vi "Permutation solution.vi"() -> ()   [LabVIEW 2018]
uses:
  ctl/Coin data--cluster.ctl
  ctl/Comparison result--enum.ctl
  <userlib>/_OpenG.lib/array/array.llb/Reverse 2D Array (Boolean)__ogtk.vi
panel:
  out "Result":string
  out "Finished message":string
  out "Goal amount":dbl=7.0 format="£%#_g"
  out "No. solutions found":i32
  out "Total left in tree":dbl format="£%.2g"
  in  "Stop":bool
  out "Total of coins selected":dbl format="£%#.2g"
  out "Coins":bool[](array[boolean])
  out "Solutions found":bool[][](array[boolean])
  # "Beer Money"
  # "Permutation Solution"
  # "What's going on?\n\nThe algorithm is doing a breadth first search of the tree.\n\nIf the result is below the goal amount, it adds it to a list to come back to later. If the result is above the goal amount, it moves the lowest value coin to the next smallest denomination.\n\nIt is seriously slow - you won't get to the end unless you have a supercomputer. Make use of the stop button.\n\nTheoretically it can check every permutation and it finds the correct solution for smaller problems."
  # "1p"
  # "2p"
  # "5p"
  # "10p"
  # "20p"
  # "50p"
  # "£1"
  # "£2"
  # "£5"
  # "£10"
  # "Link to better explanation:\n\nhttps://youtu.be/z-Rf1_xs25s"
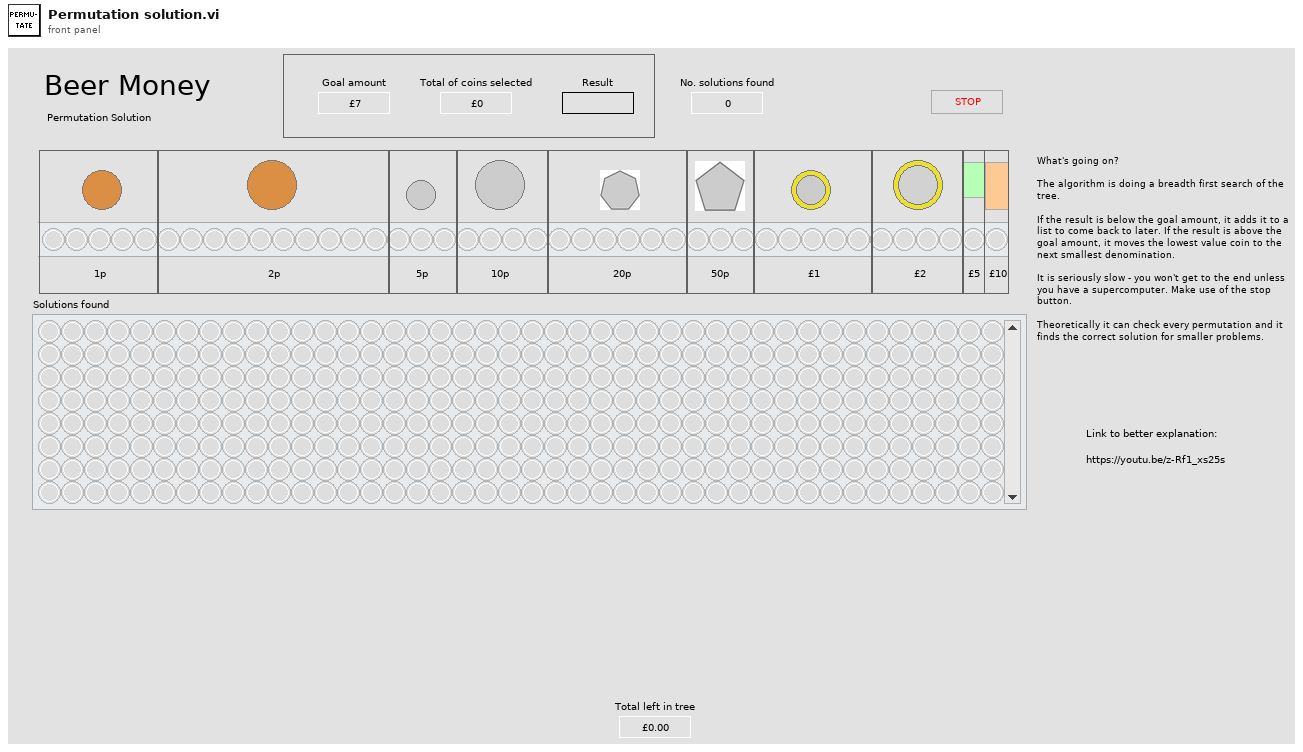
[diagram p1: front panel]
types:
  T1 = typedef "Coin data--cluster.ctl" = cluster{"Coin/note":i32, "Quantity":i32}
  T2 = cluster{"Wallet contents":T1[], "All my coins (values, £)":dbl[], "Indexes of next denom":i32[], "Wallet total (£)":dbl, "Index":i32, "Goal amount (£)":dbl, "No. coins":i32, "Coins State Cache":bool[], "Successful combos":bool[][], "'Hold' list (unexplored)":bool[][]}
  T3 = typedef "Comparison result--enum.ctl" = enum16{"Under", "Bingo!", "Over"}
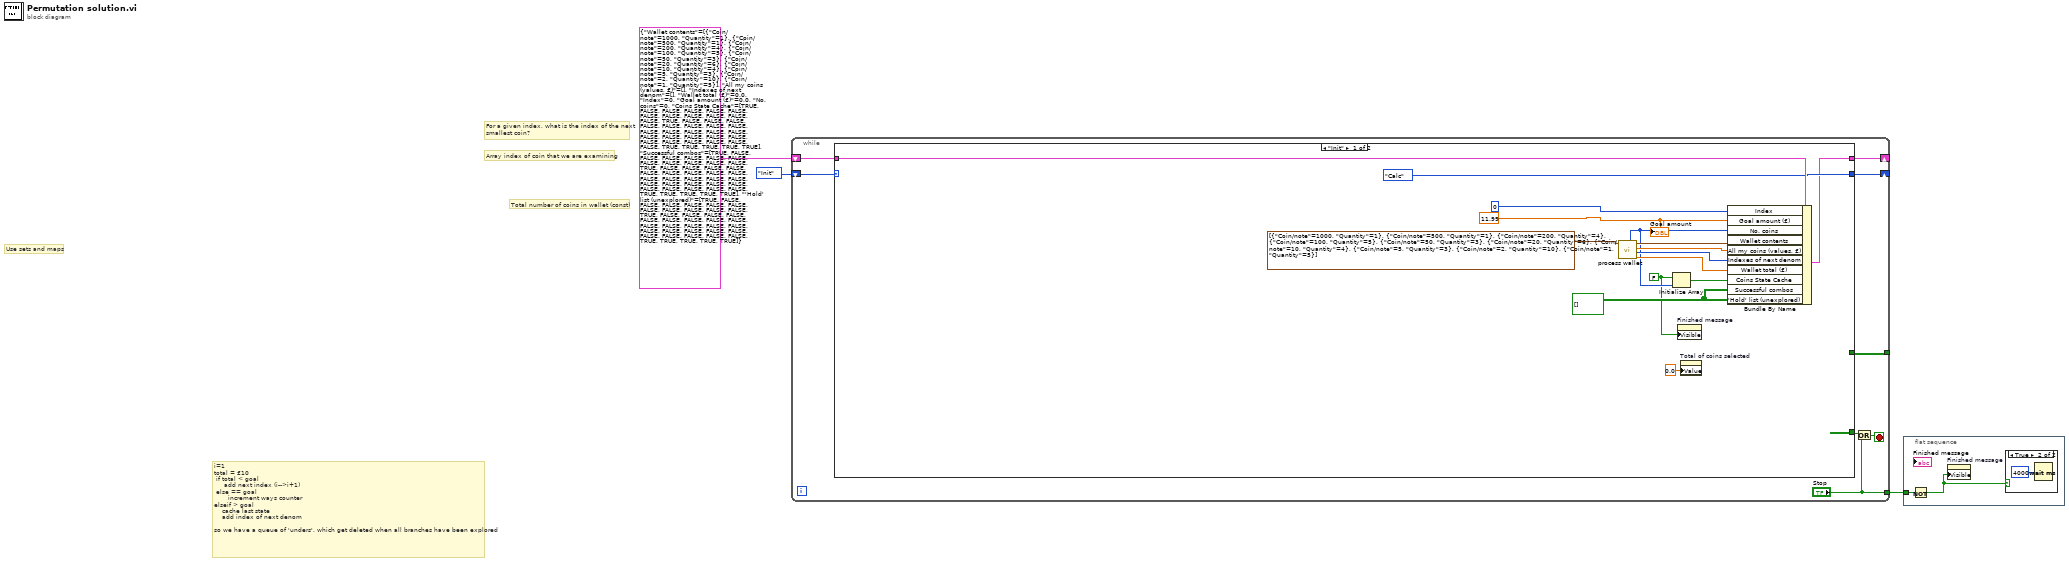
[diagram p0: block diagram]
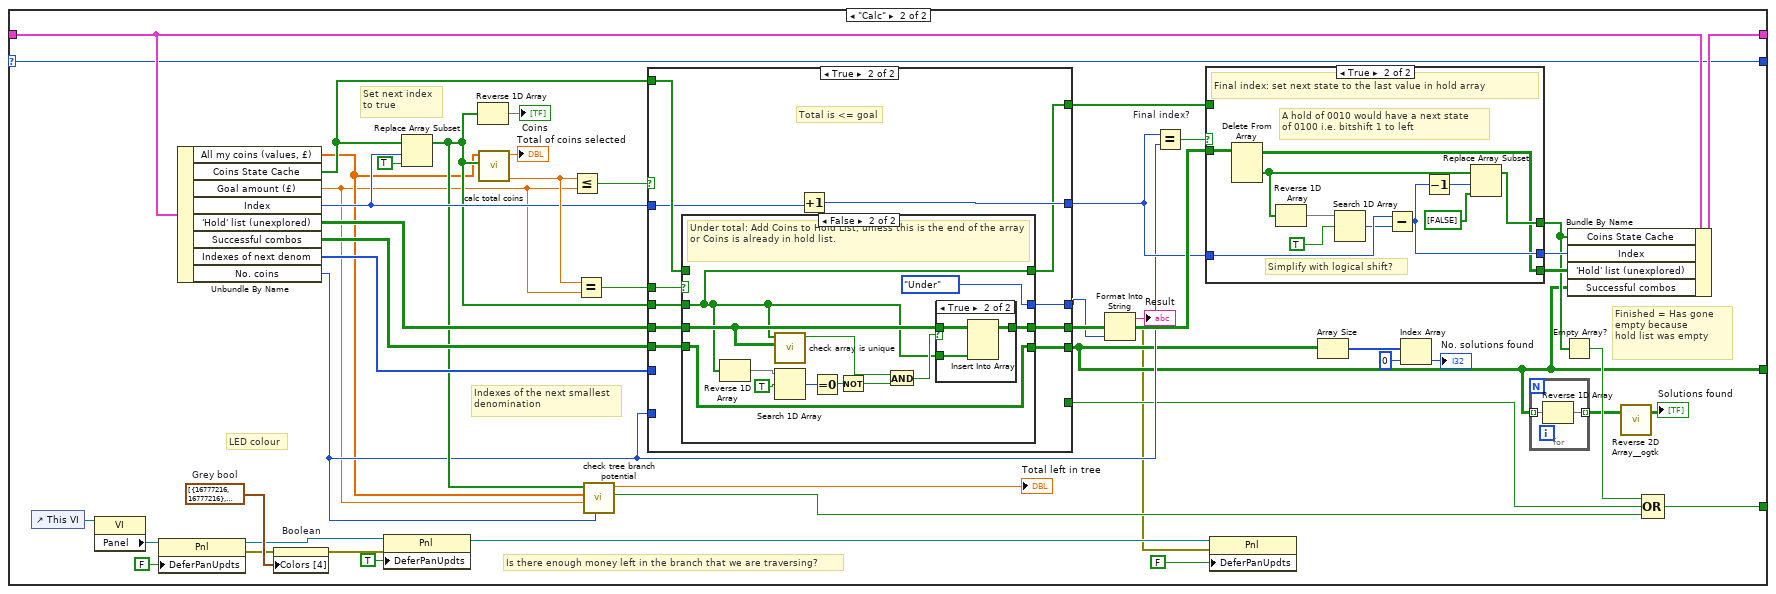
[diagram p3: hidden frame]
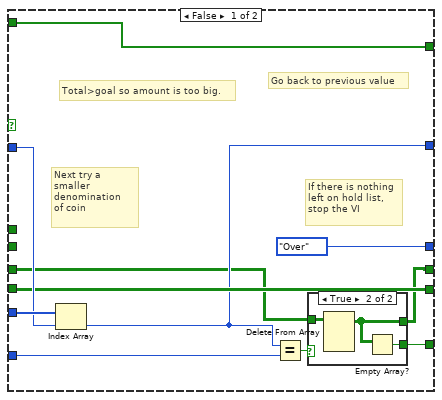
[diagram p5: hidden frame]
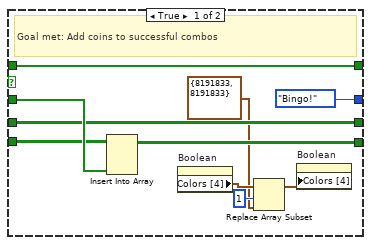
[diagram p7: hidden frame]
diagram:
  # "For a given index, what is the index of the next\nsmallest coin?"
  # "Total number of coins in wallet (const)"
  # "Array index of coin that we are examining"
  # "i=1\ntotal = £10\n if total < goal\n     add next index (i-->i+1)\n else == goal\n       increment ways counter\nelseif > goal\n    cache last state\n    add index of next denom\n\nso we have a queue of 'unders', which get deleted when all branches have been explored"
  # "Use sets and maps"
  n1 = while {
    shift-right: [w10] -> _
    shift-left: T2 {"Wallet contents"=[{"Coin/note"=1000, "Quantity"=1}, {"Coin/note"=500, "Quantity"=1}, {"Coin/note"=200, "Quantity"=4}, {"Coin/note"=100, "Quantity"=5}, {"Coin/note"=50, "Quantity"=3}, {"Coin/note"=20, "Quantity"=6}, {"Coin/note"=10, "Quantity"=4}, {"Coin/note"=5, "Quantity"=3}, {"Coin/note"=2, "Quantity"=10}, {"Coin/note"=1, "Quantity"=5}], "All my coins (values, £)"=[], "Indexes of next denom"=[], "Wallet total (£)"=0.0, "Index"=0, "Goal amount (£)"=0.0, "No. coins"=0, "Coins State Cache"=[TRUE, FALSE, FALSE, FALSE, FALSE, FALSE, FALSE, FALSE, FALSE, FALSE, FALSE, FALSE, TRUE, FALSE, FALSE, FALSE, FALSE, FALSE, FALSE, FALSE, FALSE, FALSE, FALSE, FALSE, FALSE, FALSE, FALSE, FALSE, FALSE, FALSE, FALSE, FALSE, FALSE, FALSE, FALSE, FALSE, FALSE, TRUE, TRUE, TRUE, TRUE, TRUE], "Successful combos"=[[TRUE, FALSE, FALSE, FALSE, FALSE, FALSE, FALSE, FALSE, FALSE, FALSE, FALSE, FALSE, TRUE, FALSE, FALSE, FALSE, FALSE, FALSE, FALSE, FALSE, FALSE, FALSE, FALSE, FALSE, FALSE, FALSE, FALSE, FALSE, FALSE, FALSE, FALSE, FALSE, FALSE, FALSE, FALSE, FALSE, FALSE, TRUE, TRUE, TRUE, TRUE, TRUE]], "'Hold' list (unexplored)"=[[TRUE, FALSE, FALSE, FALSE, FALSE, FALSE, FALSE, FALSE, FALSE, FALSE, FALSE, FALSE, TRUE, FALSE, FALSE, FALSE, FALSE, FALSE, FALSE, FALSE, FALSE, FALSE, FALSE, FALSE, FALSE, FALSE, FALSE, FALSE, FALSE, FALSE, FALSE, FALSE, FALSE, FALSE, FALSE, FALSE, FALSE, TRUE, TRUE, TRUE, TRUE, TRUE]]} -> [w11]
    shift-right: [w8] -> _
    shift-left: enum16{"Init", "Calc"}."Init" -> [w9]
    tunnel: [w6] -> _
    tunnel: ["Stop"] -> w1
    stop <- w5 stop-if-true
    n2 = case shown="\"Init\"" w9 {
      selector: w9 -> [_ w66]
      tunnel: w11 -> [w26 w73]
      tunnel: [w16 w74] -> w10
      tunnel: [_ w49] -> w7
      tunnel: [enum16{"Init", "Calc"}."Calc" w66] -> w8
      tunnel: [_ w43] -> w6
      frame "Init" {
        w14 = FALSE
        w23 = 11.99 ("goal amount")
        w25 = bool[][] [] ("'Hold' list (unexplored)")
        n3 = call "process wallet.vi"("Wallet contents"=T1[] [{"Coin/note"=1000, "Quantity"=1}, {"Coin/note"=500, "Quantity"=1}, {"Coin/note"=200, "Quantity"=4}, {"Coin/note"=100, "Quantity"=5}, {"Coin/note"=50, "Quantity"=3}, {"Coin/note"=20, "Quantity"=6}, {"Coin/note"=10, "Quantity"=4}, {"Coin/note"=5, "Quantity"=3}, {"Coin/note"=2, "Quantity"=10}, {"Coin/note"=1, "Quantity"=5}]) -> ("Wallet total (£)"=w19:dbl, "Indexes of next denom"=w20:i32[], "All my coins (values, £)"=w21:dbl[], "Wallet contents (dup)"=w22:T1[], "No. coins"=w15:i32)  [unwired: 6 in]
        n4 = Initialize Array(w14, w15) -> (w18:bool[])
        n5 = property on="Finished message" class="Str"("Visible"=w14) -> ()  [unwired: 2 in, 2 out]
        n6 = property on="Total of coins selected" class="DigNum (strict)"("Value"=0.0 ("Total of coins selected")) -> ()  [unwired: 2 in, 2 out]
        n7 = Bundle By Name(cluster=w26, "Index"=0, "Goal amount (£)"=w23, "No. coins"=w15, "Wallet contents"=w22, "All my coins (values, £)"=w21, "Indexes of next denom"=w20, "Wallet total (£)"=w19, "Coins State Cache"=w18, "Successful combos"=w25, "'Hold' list (unexplored)"=w25) -> (w16:T2)
        "Goal amount" <- w23
      }
      frame "Calc" {
        w39 = cluster{u32, u32}[] [{16777216, 16777216}, {8026746, 8026746}, {16777216, 16777216}, {4095788, 4095788}]  # Grey bool
        # "LED colour"
        # "Indexes of the next smallest\ndenomination"
        # "Is there enough money left in the branch that we are traversing?"
        # "Set next index to true"
        # "Finished = Has gone empty because\nhold list was empty"
        n8 = control-ref of="This VI"() -> (w37:refnum<vi>)
        n9 = property class="VI"(reference=w37) -> ("Panel"=w36:refnum<vi>)  [unwired: 1 in, 2 out]
        n10 = property class="Pnl"(reference=w36, "DeferPanUpdts"=FALSE ("Defer Panel Updates")) -> (reference out=w33:refnum<vi>, error out=w30:errorcluster)  [unwired: 1 in]
        n11 = Unbundle By Name(w73) -> ("All my coins (values, £)"=w52:dbl[], "Coins State Cache"=w55:bool[], "Goal amount (£)"=w50:dbl, "Index"=w62:i32, "'Hold' list (unexplored)"=w69:bool[][], "Successful combos"=w68:bool[][], "Indexes of next denom"=w67:i32[], "No. coins"=w53:i32)
        n12 = property on="Boolean" class="Bool (strict)"(error in=w30, "Colors [4]"=w39) -> (error out=w32:errorcluster)  [unwired: 1 in, 1 out]
        n13 = property class="Pnl"(reference=w33, error in=w32, "DeferPanUpdts"=TRUE ("Defer Panel Updates")) -> (reference out=w29:refnum<vi>)  [unwired: 1 out]
        n14 = Replace Array Subset(array=w55, new element=TRUE ("new element/subarray"), index=w62) -> (w54:bool[])
        n15 = Reverse 1D Array(array=w54) -> (reversed array=→"Coins":bool[])
        n16 = call "calc total coins.vi"("Coins"=w54, "All my coins"=w52) -> ("Total (£)"=w71:dbl)  [unwired: 9 in]
        "Total of coins selected" <- w71
        n17 = Less Or Equal?(x=w71, y=w50) -> (x <= y?=w72:bool)
        n18 = Equal?(x=w71, y=w50) -> (x = y?=w70:bool)
        n19 = call "check tree branch potential.vi"("No. coins"=w53, "Goal amount"=w50, "All my coins"=w52, "Coins State Cache"=w54) -> ("Stop?"=w48:bool, "Total (£)"=→"Total left in tree":dbl)  [unwired: 6 in]
        n20 = case "Goal amount exceeded?" shown="True" w72 {
          tunnel: w70 -> [_ w106]
          tunnel: w62 -> [w100 w107]
          tunnel: [w96 w116] -> w59
          tunnel: w54 -> [_ w112]
          tunnel: w69 -> [w95 w115]
          tunnel: w68 -> [w99 w114]
          tunnel: [w99 w113] -> w43
          tunnel: [w94 w111] -> w63
          tunnel: w67 -> [w101 _]
          tunnel: [w92 w109] -> w64
          tunnel: w53 -> [w97 _]
          tunnel: [w93 _] -> w47
          tunnel: w55 -> [w92 w108]
          tunnel: [Comparison_result--enum."Over" ("Total") w110] -> w35
          frame False {
            # "If there is nothing\nleft on hold list,\nstop the VI"
            # "Go back to previous value"
            # "Next try a smaller denomination\nof coin"
            # "Total>goal so amount is too big."
            n21 = Index Array(array=w101, index=w100) -> (element=w96:i32)
            n22 = Equal?(x=w96, y=w97) -> (x = y?=w98:bool)
            n23 = case shown="True" w98 {
              tunnel: [w102 w104] -> w94
              tunnel: w95 -> [w102 w105]
              tunnel: [_ w103] -> w93
              frame False {
              }
              frame True {
                n24 = Delete From Array(array=w105) -> (array with subset deleted=w104:bool[][])  [unwired: 3 in, 1 out]
                n25 = Empty Array?(array=w104) -> (empty?=w103:bool)
              }
            }
          }
          frame True {
            # "Total is <= goal"
            n26 = case shown="False" w106 {
              tunnel: w115 -> [w123 w135]
              tunnel: w114 -> [w125 w137]
              tunnel: [w124 w137] -> w113
              tunnel: w112 -> [w126 w127]
              tunnel: [w123 w138] -> w111
              tunnel: [Comparison_result--enum."Bingo!" ("Total") Comparison_result--enum."Under" ("Total")] -> w110
              tunnel: [w121 w127] -> w109
              tunnel: w108 -> [w121 _]
              frame True {
                # "Goal met: Add coins to successful combos"
                n27 = Insert Into Array(array=w125, new element=w126) -> (w124:bool[][])  [unwired: 2 in]
                n28 = property on="Boolean" class="Bool (strict)"() -> ("Colors [4]"=w120:cluster{u32, u32}[])  [unwired: 2 in, 2 out]
                n29 = Replace Array Subset(array=w120, new element=cluster{u32, u32} {8191833, 8191833} ("new element/subarray"), index=1) -> (w118:cluster{u32, u32}[])
                n30 = property on="Boolean" class="Bool (strict)"("Colors [4]"=w118) -> ()  [unwired: 2 in, 2 out]
              }
              frame False {
                # "Under total: Add Coins to Hold List, unless this is the end of the array or Coins is already in hold list."
                n31 = Reverse 1D Array(array=w127) -> (reversed array=w131:bool[])
                n32 = call "check array is unique.vi"("'Hold' list"=w135, "Coins State Cache"=w127) -> ("Is unique?"=w134:bool)  [unwired: 9 in]
                n33 = Search 1D Array(1D array=w131, element=TRUE) -> (index of element=w130:i32)  [unwired: 1 in]
                n34 = Equal To 0?(x=w130) -> (x = 0?=w129:bool)
                n35 = Not(x=w129) -> (.not. x?=w128:bool)
                n36 = And(x=w134, y=w128) -> (x .and. y?=w133:bool)
                n37 = case shown="True" w133 {
                  tunnel: [w139 w142] -> w138
                  tunnel: w135 -> [w139 w141]
                  tunnel: w127 -> [_ w140]
                  frame False {
                  }
                  frame True {
                    n38 = Insert Into Array(array=w141, new element=w140) -> (w142:bool[][])  [unwired: 2 in]
                  }
                }
              }
            }
            n39 = Increment(x=w107) -> (x+1=w116:i32)
          }
        }
        n40 = Format Into String(w35) -> (resulting string=→"Result":string, error out=w27:errorcluster)  [unwired: 3 in]
        n41 = Equal? "Final index?"(x=w59, y=w53) -> (x = y?=w65:bool)
        n42 = case shown="True" w65 {
          tunnel: w63 -> [w78 w86]
          tunnel: [w79 w88] -> w56
          tunnel: w64 -> [w79 _]
          tunnel: [w78 w87] -> w57
          tunnel: [w77 w89] -> w60
          tunnel: w59 -> [w77 w90]
          frame False {
            # "Not final index - do nothing"
          }
          frame True {
            # "Simplify with logical shift?"
            # "A hold of 0010 would have a next state\nof 0100 i.e. bitshift 1 to left"
            # "Final index: set next state to the last value in hold array"
            n43 = Delete From Array(array=w86) -> (deleted portion=w82:bool[], array with subset deleted=w87:bool[][])  [unwired: 3 in]
            n44 = Reverse 1D Array(array=w82) -> (reversed array=w83:bool[])
            n45 = Search 1D Array(1D array=w83, element=TRUE) -> (index of element=w80:i32)  [unwired: 1 in]
            n46 = Subtract(x=w90, y=w80) -> (x-y=w89:i32)
            n47 = Decrement(x=w89) -> (x-1=w81:i32)
            n48 = Replace Array Subset(array=w82, new element=bool[] [FALSE] ("new element/subarray"), index=w81) -> (w88:bool[])
          }
        }
        n49 = property class="Pnl"(reference=w29, error in=w27, "DeferPanUpdts"=FALSE ("Defer Panel Updates")) -> ()  [unwired: 2 out]
        n50 = Array Size(array=w43) -> (size(s)=w45:i32[])
        n51 = Index Array(array=w45, index=0) -> (element=→"No. solutions found":i32)
        n52 = for {
          tunnel: w43 -> [w76] mode=indexing
          tunnel: [w75] -> w41 mode=indexing
          n53 = Reverse 1D Array(array=w76) -> (reversed array=w75:bool[])
        }
        n54 = Empty Array?(array=w56) -> (empty?=w46:bool)
        n55 = Bundle By Name(cluster=w73, "Coins State Cache"=w56, "Index"=w60, "'Hold' list (unexplored)"=w57, "Successful combos"=w43) -> (w74:T2)
        n56 = call-poly <userlib>:"Reverse 2D Array__ogtk.vi"("Array"=w41) -> ("Reversed Array"=→"Solutions found":bool[][])  [unwired: 2 in]
        n57 = Compound Arithmetic op=OR(w46, w47, w48) -> (w49:bool)
      }
    }
    n58 = Or(x=w7, y="Stop") -> (x .or. y?=w5:bool)
  }
  n59 = flat-sequence {
    tunnel: w1 -> [w144]
    frame #0 {
      n60 = Not(x=w144) -> (.not. x?=w143:bool)
      n61 = property on="Finished message" class="Str"("Visible"=w143) -> ()  [unwired: 2 in, 2 out]
      n62 = case shown="True" w143 {
        frame False {
        }
        frame True {
          n63 = Wait (ms)(milliseconds to wait=u32 4000) -> ()  [unwired: 1 out]
        }
      }
    }
  }
